vi "Set Busy Indicator.vi"(7 "Busy":bool, 11 "error in (no error)":errorcluster) -> (3 "error out":errorcluster)   [LabVIEW 2023]
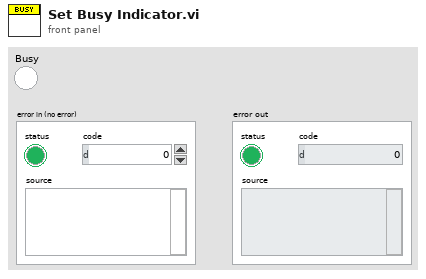
[diagram p1: front panel]
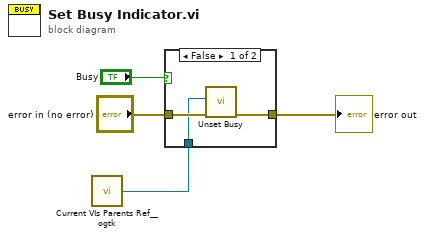
[diagram p0: block diagram]
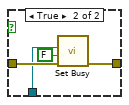
[diagram p2: hidden frame]
diagram:
  n1 = call <userlib>:"Current VIs Parents Ref__ogtk.vi"() -> ("Calling VI's Reference"=w1:refnum<vi>)  [unwired: 2 in]
  n2 = case shown="False" "Busy" {
    tunnel: [w6 w11] -> w4
    tunnel: "error in (no error)" -> [w7 w10]
    tunnel: w1 -> [w5 w8]
    frame False {
      n3 = call <vilib>:"Unset Busy.vi"("error in (no error)"=w7, "VI reference (current VI)"=w5) -> ("error out"=w6:errorcluster)  [unwired: 9 in]
    }
    frame True {
      n4 = call <vilib>:"Set Busy.vi"("error in (no error)"=w10, "disable click? (T)"=FALSE, "VI reference (current VI)"=w8) -> ("error out"=w11:errorcluster)  [unwired: 7 in, 1 out]
    }
  }
  "error out" <- w4
